vi "test.vi"() -> ()   [LabVIEW 2025, in "mass-spring-damper.lvclass"]
uses:
  mass-spring-damper.lvclass
  mass-spring-damper.lvclass/mass-spring-damper.ctl
  Dynamic-System/Dynamic-System.lvclass
  C:/Users/Tyson.Grover/Desktop/Repositories/dynamic-systems/Classes/Dynamic-System/Dynamic-System.lvclass
  C:/Users/Tyson.Grover/Desktop/Repositories/dynamic-systems/Classes/mass-spring-damper/mass-spring-damper.lvclass
  Dynamic-System/dynamic system selection.ctl
panel:
  in  "Config Path":path
  in  "Dynamic System":T1
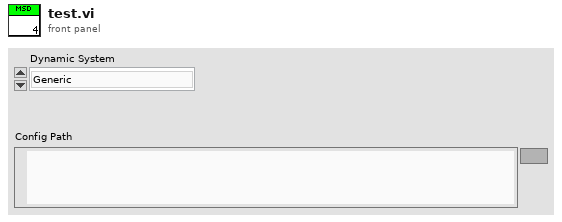
[diagram p1: front panel]
types:
  T1 = typedef "dynamic system selection.ctl" = enum16{"Generic", "Mass Spring Damper", "Liquid Tank", "RLC Circuit"}
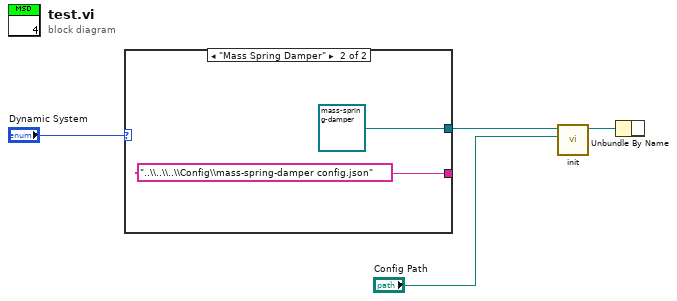
[diagram p0: block diagram]
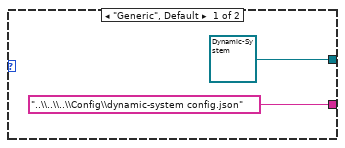
[diagram p2: hidden frame]
diagram:
  n1 = case shown="\"Mass Spring Damper\"" "Dynamic System" {
    tunnel: [refnum<class "Dynamic-System.lvclass"> refnum ("Dynamic-System.lvclass") refnum<class "mass-spring-damper.lvclass"> refnum ("mass-spring-damper.lvclass")] -> w4
    tunnel: ["..\\..\\..\\Config\\dynamic-system config.json" "..\\..\\..\\Config\\mass-spring-damper config.json"] -> _
    frame "Generic", Default {
    }
    frame "Mass Spring Damper" {
    }
  }
  n2 = call-dynamic "init.vi"("Config Path"="Config Path", "Dynamic-System in"=w4) -> ("Dynamic-System out"=w1:refnum<class "Dynamic-System.lvclass">)  [unwired: 8 in, 1 out]
  n3 = Unbundle By Name(w1) -> ()  [unwired: 1 out]
